vi "Packetize.vi"(8 "Error In":errorcluster, 9 "ARGS":u8[](array[numeric]), 10 "CMD":u16, 11 "LINX Device Config":T1) -> (0 "Error Out":errorcluster, 2 "Packet":string, 3 "LINX Decice Config":T1)   [LabVIEW 2011, in "LVH-LINX.lvlib"]
doc: "This VI takes a LINX command and arguments and builds a LINX packet."
uses:
  LVH-LINX.lvlib
  Type Defs/LINX Device Config.ctl
  Type Defs/Interface.ctl
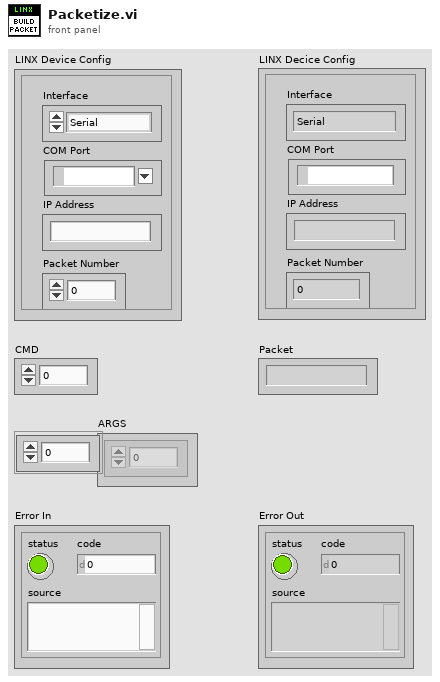
[diagram p1: front panel]
types:
  T1 = typedef "LVH-LINX.lvlib/LINX Device Config.ctl" = cluster{"Interface":T2, "COM Port":refnum<visa-resource-name>, "IP Address":string, "Packet Number":u16}
  T2 = typedef "LVH-LINX.lvlib/Interface.ctl" = enum16{"Serial", "TCP"}
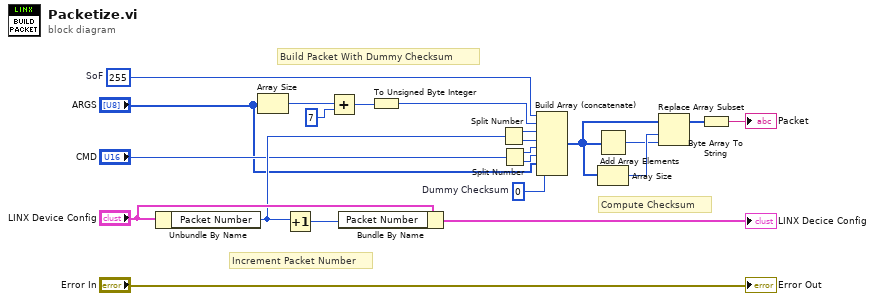
[diagram p0: block diagram]
diagram:
  w8 = u8 0  # Dummy Checksum
  w18 = u8 255  # SoF
  # "Increment Packet Number"
  # "Build Packet With Dummy Checksum"
  # "Compute Checksum"
  n1 = Unbundle By Name("LINX Device Config") -> ("Packet Number"=w15:u16)
  n2 = Array Size(array="ARGS") -> (size(s)=w20:i32)
  n3 = Increment(x=w15) -> (x+1=w21:u16)
  n4 = Add(x=w20, y=7) -> (x+y=w17:i32)
  n5 = Bundle By Name(cluster="LINX Device Config", "Packet Number"=w21) -> (→"LINX Decice Config":T1)
  n6 = To Unsigned Byte Integer(number=w17) -> (unsigned 8bit integer=w16:u8)
  n7 = Split Number(x=w15) -> (hi(x)=w14:u8, lo(x)=w13:u8)
  n8 = Split Number(x="CMD") -> (hi(x)=w12:u8, lo(x)=w11:u8)
  n9 = Build Array (concatenate)(w18, w16, w14, w13, w12, w11, "ARGS", w8) -> (w6:u8[])
  n10 = Add Array Elements(numeric array=w6) -> (sum=w5:u8)
  n11 = Array Size(array=w6) -> (size(s)=w7:i32)
  n12 = Replace Array Subset(array=w6, new element=w5, index=w7) -> (w2:u8[])
  n13 = Byte Array To String(unsigned byte array=w2) -> (string=→"Packet":string)
  "Error Out" <- "Error In"
